vi "raceCondition.vi"() -> ()   [LabVIEW 2020]
panel:
  out "Total":i32
  out "L2":i32
  out "L1":i32
  in  "stop":bool
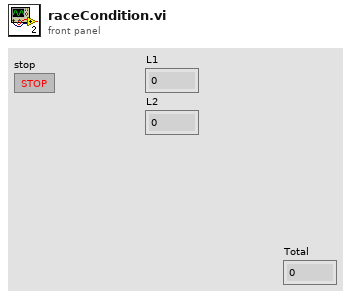
[diagram p1: front panel]
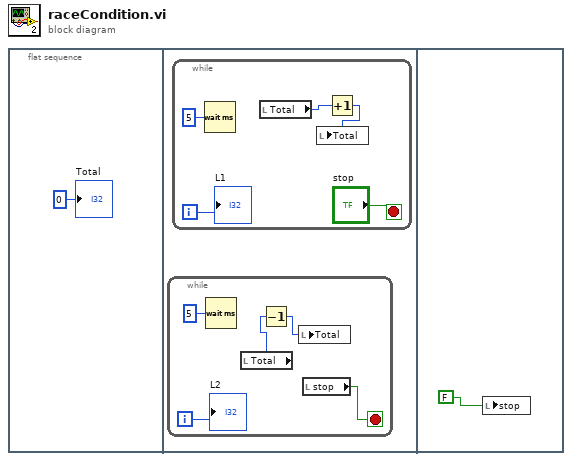
[diagram p0: block diagram]
diagram:
  n1 = flat-sequence {
    frame #0 {
      "Total" <- 0 ("Total")
    }
    frame #1 {
      n2 = while {
        i -> [w10]
        stop <- w11 stop-if-true
        n3 = Wait (ms)(milliseconds to wait=u32 5) -> ()  [unwired: 1 out]
        n4 = local read "Total"() -> (w7:i32)
        n5 = Decrement(x=w7) -> (x-1=w8:i32)
        n6 = local write "Total"(w8) -> ()
        n7 = local read "stop"() -> (w11:bool)
        "L2" <- w10
      }
      n8 = while {
        i -> [w5]
        stop <- "stop" stop-if-true
        n9 = Wait (ms)(milliseconds to wait=u32 5) -> ()  [unwired: 1 out]
        n10 = local read "Total"() -> (w3:i32)
        n11 = Increment(x=w3) -> (x+1=w2:i32)
        n12 = local write "Total"(w2) -> ()
        "L1" <- w5
      }
    }
    frame #2 {
      n13 = local write "stop"(FALSE) -> ()
    }
  }
